vi "example.vi"   [LabVIEW 2017]
uses:
  vs-tree-utility.lvlib
types:
  T1 = cluster{"Type":enum16{"Channel", "Waveform", "Section"}, "Parameters":variant, "Show Only Visible?":bool}[]
  T2 = cluster{"Allow Multi Select":bool, "Use Checkboxes":bool, "Text Prompt":string}
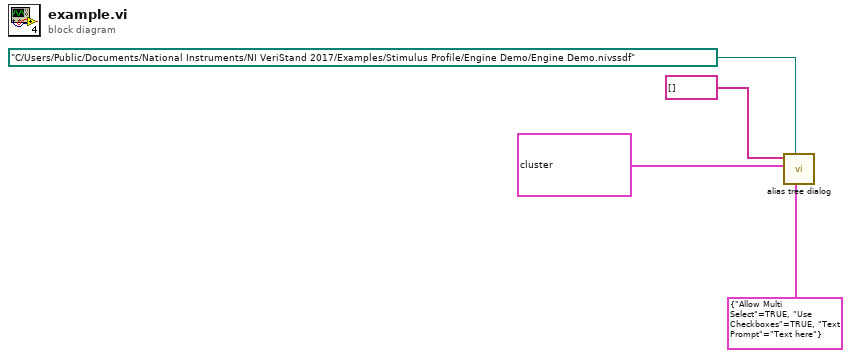
[diagram p0: block diagram]
diagram:
  n1 = call "alias tree dialog.vi"("Tree Config"=T2 {"Allow Multi Select"=TRUE, "Use Checkboxes"=TRUE, "Text Prompt"="Text here"}, "SDF Path"=path "C:/Users/Public/Documents/National Instruments/NI VeriStand 2017/Examples/Stimulus Profile/Engine Demo/Engine Demo.nivssdf", "Filter Config"=T1 [{"Type"=enum."Channel", "Parameters"=variant, "Show Only Visible?"=FALSE}], "Current Selection"=string[] []) -> ()  [unwired: 6 in, 2 out]
